vi "[Global] ExtractedProcessImage.vi"() -> ()   [LabVIEW 2019]
panel:
  out "ExtractedProcessImageArray":string[](array[string])=["ExtractedProcessedImage0", "ExtractedProcessedImage1", "ExtractedProcessedImage2", "ExtractedProcessedImage3", "ExtractedProcessedImage4", "ExtractedProcessedImage5", "ExtractedProcessedImage6", "ExtractedProcessedImage7"]
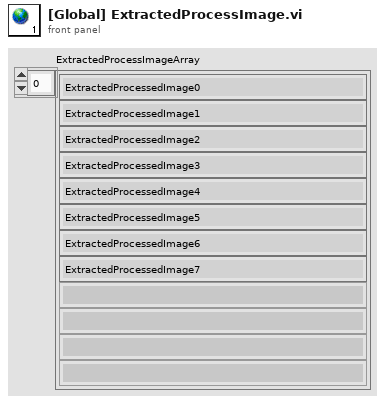
[diagram p1: front panel]
diagram:
